vi "fpga4.vi"() -> ()   [LabVIEW 2015]
uses:
  <vilib>/LabVIEW Targets/FPGA/RIO/nicrio_985x_controls.llb/CAN_IO_Frame Cluster.ctl
  <vilib>/LabVIEW Targets/FPGA/RIO/nicrio_985x_controls.llb/CAN_IO_Frame Type.ctl
  <vilib>/rvi/Emulation/niFpgaGetClockAttributes.vi
  <vilib>/rvi/Emulation/niFpgaSctlEmulationGetInTimedLoop.vi
  <vilib>/rvi/Emulation/niFpgaEmulationReportErrorSimple.vi
  <vilib>/rvi/eio/common/nirviEmuTemplateMethod_errors.vi
  <vilib>/rvi/Emulation/niFpgaCriticalErrorInLSC.vi
  <vilib>/eio/EIONode/EIONode.xnode
  <vilib>/eio/EIOMethodNode/EIOMethodNode.xnode
panel:
  out "can 316":u8[](array[numeric])
  out "can 690":u8[](array[numeric])
  out "can 545":u8[](array[numeric])
  out "can 4F0":u8[](array[numeric])
  out "can 4B0":u8[](array[numeric])
  out "can 43F":u8[](array[numeric])
  out "can 392":u8[](array[numeric])
  out "can 329":u8[](array[numeric])
  out "can 220":u8[](array[numeric])
  out "can data":u32[](array[numeric])
  out "can 164":u8[](array[numeric])
  in  "Mod4/CAN1 input":T1={"timestamp high"=0, "timestamp low"=0, "identifier"=0, "type"=enum."Data Frame", "info A"=0, "info B"=0, "data length"=0, "data"=[0, 0, 0, 0, 0, 0, 0, 0]} {"identifier" format="%x"; "timestamp high" format="%08x"; "timestamp low" format="%08x"; "data" format="%.0x"}
  in  "send can":bool
  out "Mod4/CAN1 read":T1={"timestamp high"=0, "timestamp low"=0, "identifier"=0, "type"=enum."Data Frame", "info A"=0, "info B"=0, "data length"=0, "data"=[0, 0, 0, 0, 0, 0, 0, 0]} {"identifier" format="%x"; "timestamp high" format="%08x"; "timestamp low" format="%08x"; "data" format="%.0x"}
  out "can0 error out1":errorcluster
  out "can0 error out":errorcluster
  out "m 760":u8[](array[numeric])
  out "m 729":u8[](array[numeric])
  out "m 728":u8[](array[numeric])
  out "m 727":u8[](array[numeric])
  out "m 726":u8[](array[numeric])
  out "m 725":u8[](array[numeric])
  out "m 724":u8[](array[numeric])
  out "m 723":u8[](array[numeric])
  out "m 722":u8[](array[numeric])
  out "m 721":u8[](array[numeric])
  out "m 720":u8[](array[numeric])
  out "m 711":u8[](array[numeric])
  out "m 710":u8[](array[numeric])
  out "m 700":u8[](array[numeric])
  out "Mod4/CAN0":T1={"timestamp high"=0, "timestamp low"=0, "identifier"=0, "type"=enum."Data Frame", "info A"=0, "info B"=0, "data length"=0, "data"=[0, 0, 0, 0, 0, 0, 0, 0]} {"identifier" format="%x"; "timestamp high" format="%08x"; "timestamp low" format="%08x"; "data" format="%.0x"}
  out "brk enc":u8
  in  "baud rate":i32(ring)=4 items=["300", "1200", "2400", "4800", "9600", "14400", "19200", "28800", "38400", "57600", "115200", "230400"]
  in  "B Pwm":u16=1500
  in  "T Pwm":u16=1500
  in  "S Pwm 1":u16=1500
  in  "S Pwm 2":u16=1500
  out "Auto":bool
  out "Run":bool
  in  "Solenoid":bool
  in  "Buzz":bool
  out "T Lim":bool
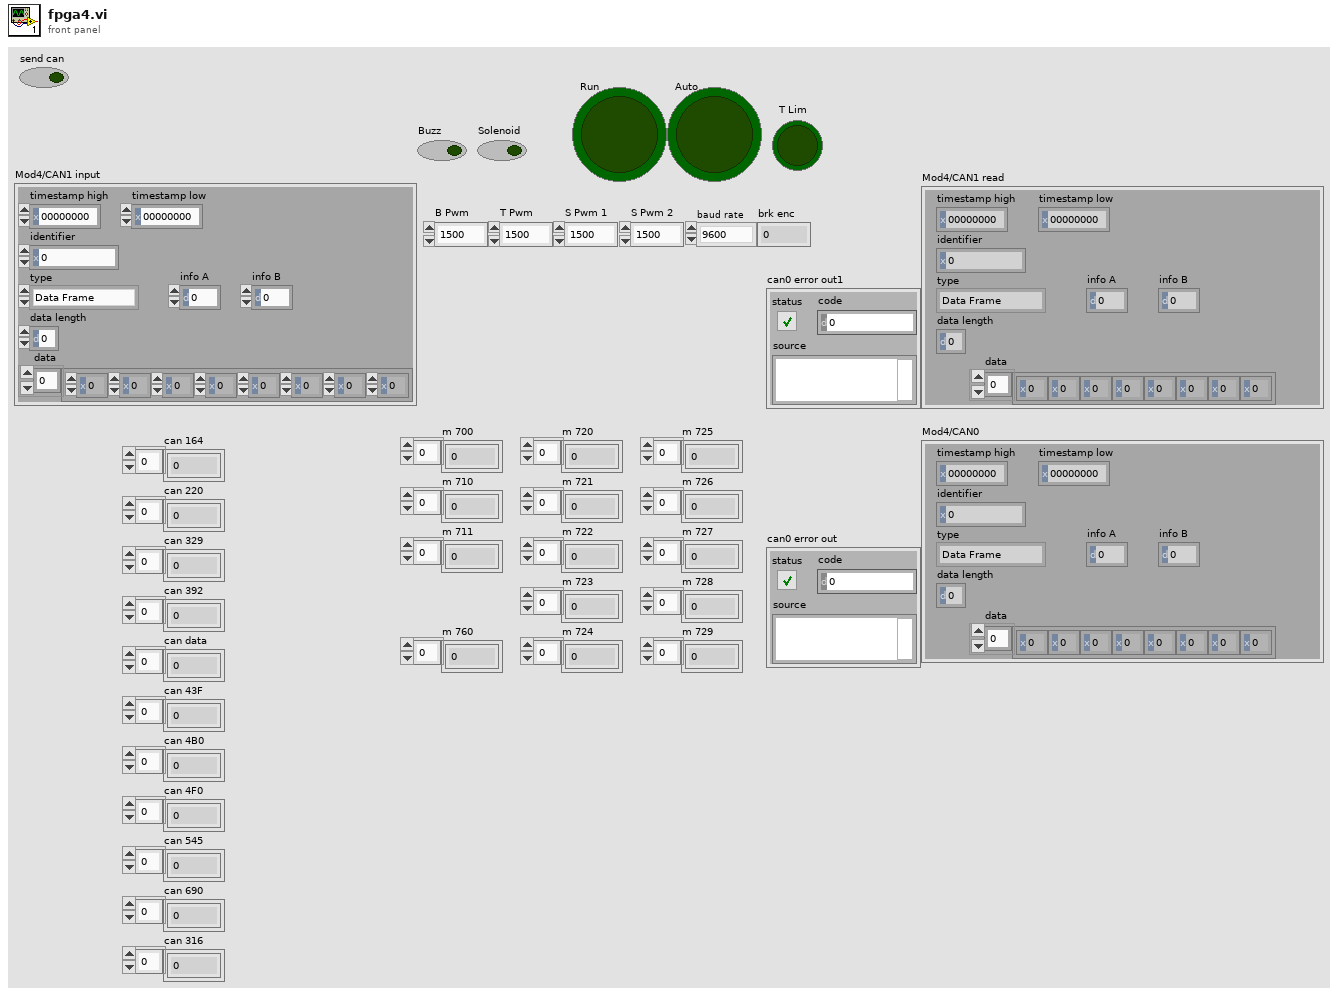
[diagram p1: front panel]
types:
  T1 = typedef "CAN_IO_Frame Cluster.ctl" = cluster{"timestamp high":u32, "timestamp low":u32, "identifier":u32, "type":T2, "info A":u8, "info B":u8, "data length":u8, "data":u8[]}
  T2 = typedef "CAN_IO_Frame Type.ctl" = enum8{"Data Frame", "Remote Frame", "(reserved)", "(reserved) ", "(reserved)  ", "(reserved)   ", "Bus Error", "Transceiver Fault"}
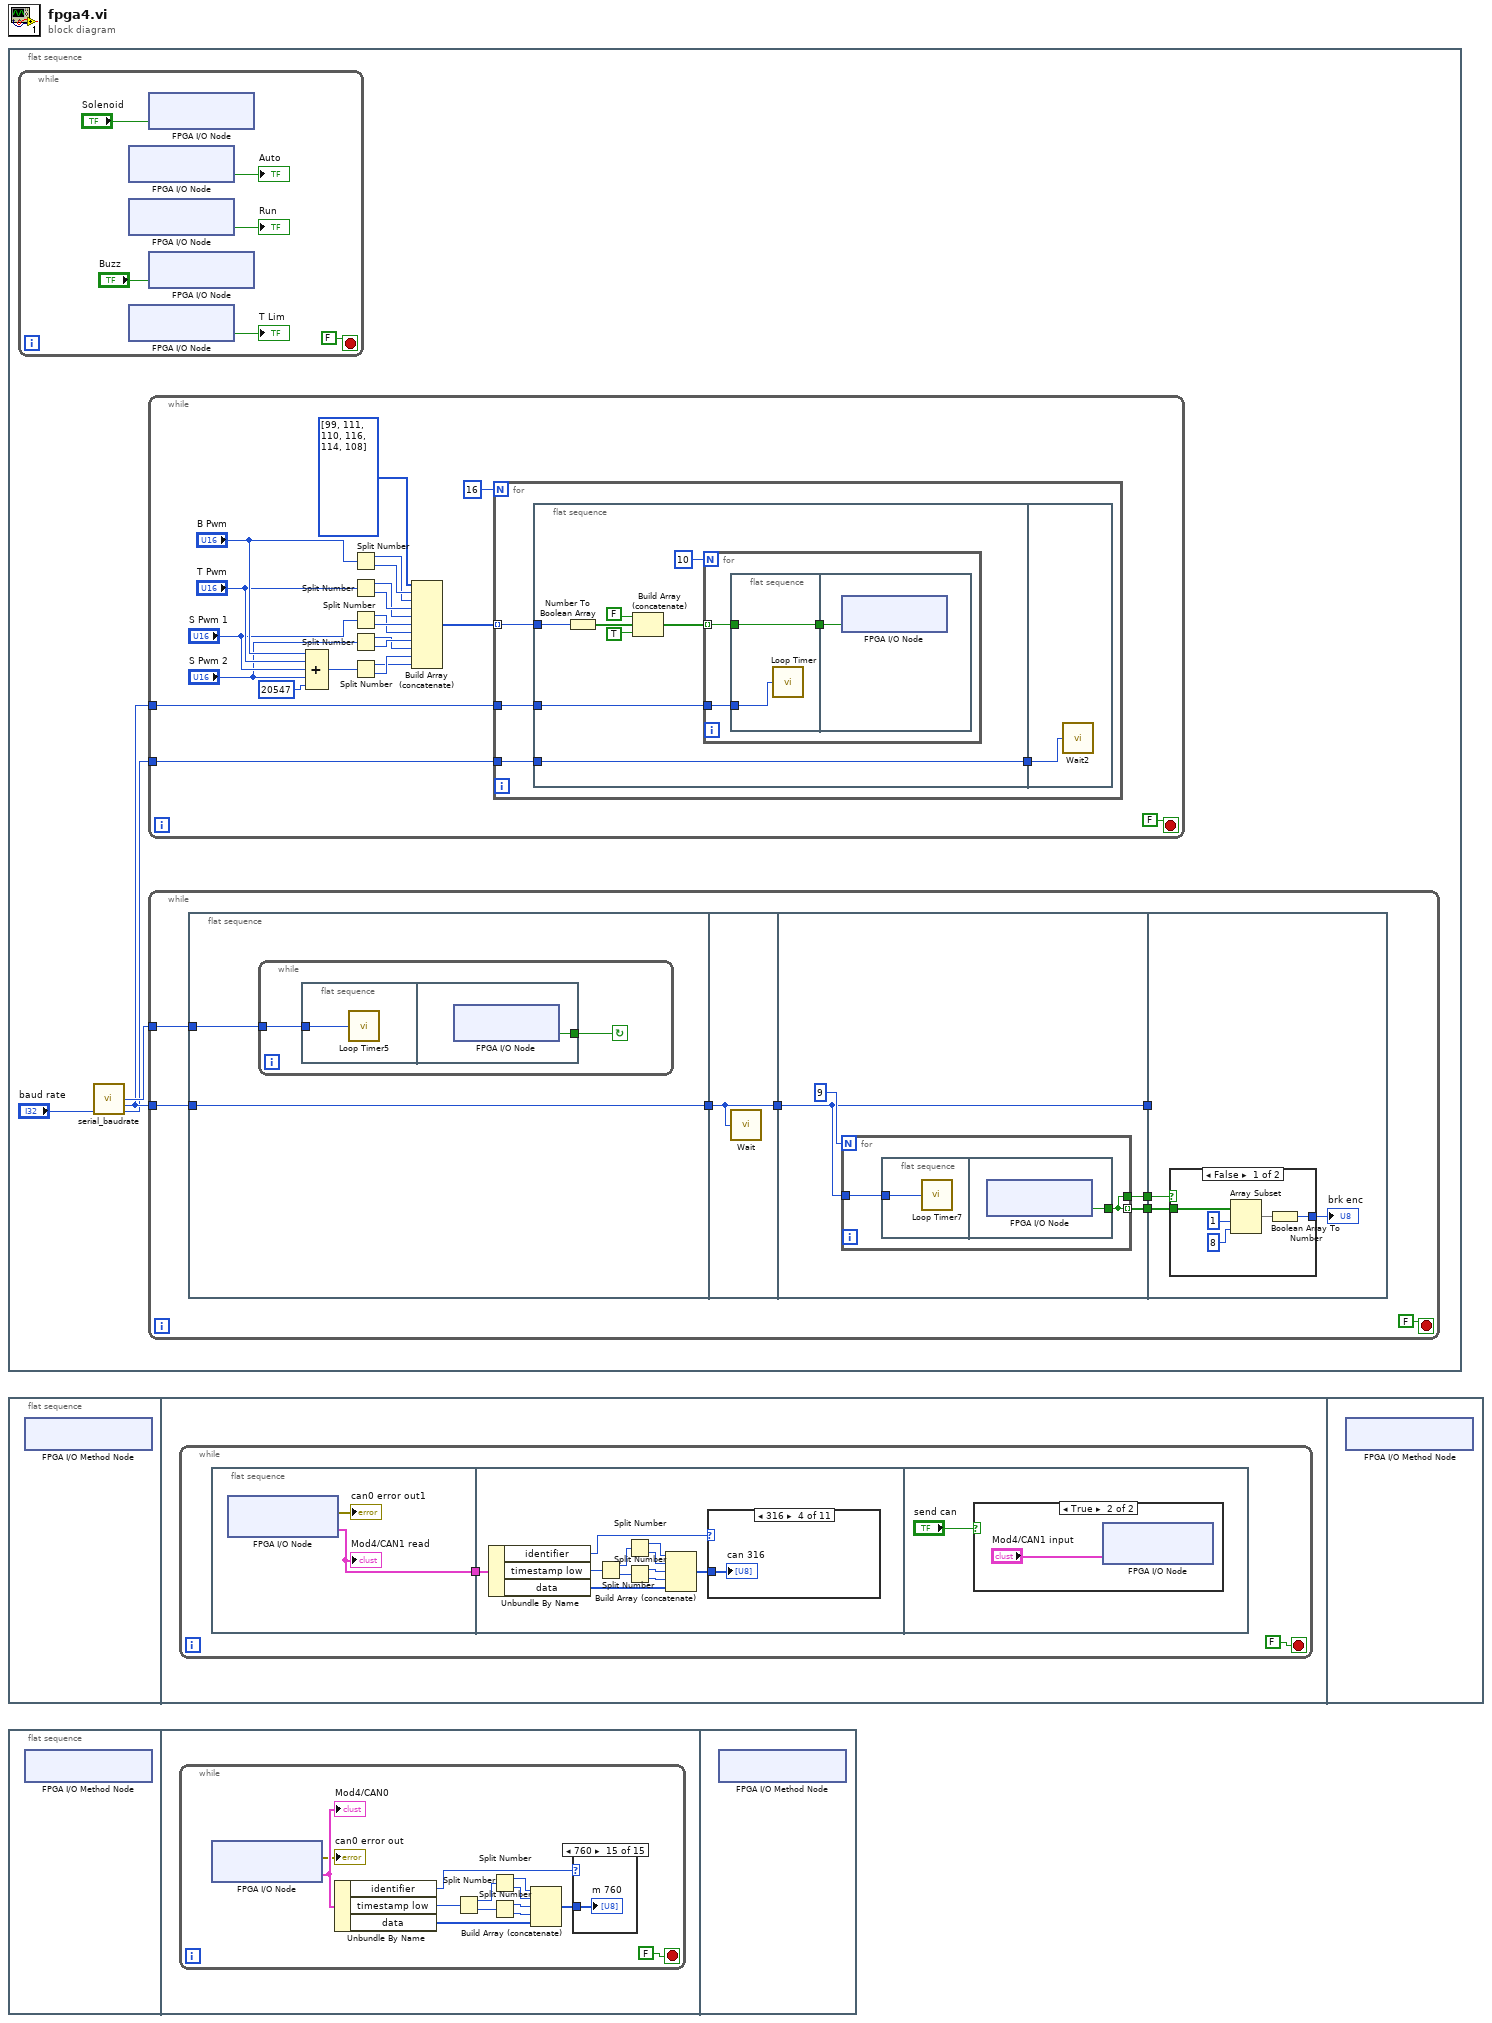
[diagram p0: block diagram]
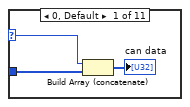
[diagram p2: hidden frame]
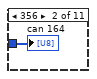
[diagram p3: hidden frame]
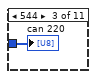
[diagram p4: hidden frame]
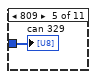
[diagram p5: hidden frame]
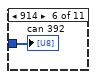
[diagram p6: hidden frame]
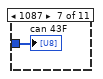
[diagram p7: hidden frame]
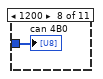
[diagram p8: hidden frame]
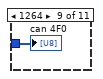
[diagram p9: hidden frame]
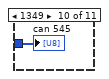
[diagram p10: hidden frame]
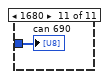
[diagram p11: hidden frame]
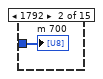
[diagram p14: hidden frame]
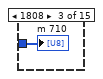
[diagram p15: hidden frame]
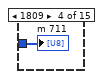
[diagram p16: hidden frame]
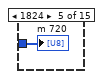
[diagram p17: hidden frame]
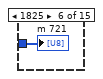
[diagram p18: hidden frame]
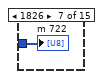
[diagram p19: hidden frame]
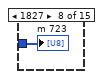
[diagram p20: hidden frame]
diagram:
  n1 = flat-sequence {
    frame #0 {
      n2 = while {
        stop <- FALSE stop-if-true
        n3 = xnode "FPGA I/O Node"() -> ("Mod3/DIO0"=→"Auto":bool)  [unwired: 1 in, 1 out]
        n4 = xnode "FPGA I/O Node"() -> ("Mod3/DIO3"=→"Run":bool)  [unwired: 1 in, 1 out]
        n5 = xnode "FPGA I/O Node"() -> ("Mod3/DIO2"=→"T Lim":bool)  [unwired: 1 in, 1 out]
        n6 = xnode "FPGA I/O Node"("Mod3/DIO4"="Solenoid") -> ()  [unwired: 1 in, 1 out]
        n7 = xnode "FPGA I/O Node"("Mod3/DIO5"="Buzz") -> ()  [unwired: 1 in, 1 out]
      }
      n8 = call "serial_baudrate.vi"("baud rate"="baud rate") -> ("tick/2 every bit"=w3:u32, "tick every bit"=w2:u32, "tick after stop bit"=w1:u32)  [unwired: 12 in]
      n9 = while {
        tunnel: w2 -> [w6]
        tunnel: w1 -> [w5]
        stop <- FALSE stop-if-true
        n10 = Compound Arithmetic op=ADD("B Pwm", "T Pwm", "S Pwm 1", "S Pwm 2", u16 20547 ("value")) -> (w11:u16)
        n11 = Split Number(x="B Pwm") -> (hi(x)=w24:u8, lo(x)=w25:u8)
        n12 = Split Number(x="T Pwm") -> (hi(x)=w22:u8, lo(x)=w23:u8)
        n13 = Split Number(x="S Pwm 1") -> (hi(x)=w20:u8, lo(x)=w21:u8)
        n14 = Split Number(x="S Pwm 2") -> (hi(x)=w18:u8, lo(x)=w19:u8)
        n15 = Split Number(x=w11) -> (hi(x)=w9:u8, lo(x)=w10:u8)
        n16 = Build Array (concatenate)(u8[] [99, 111, 110, 116, 114, 108] ("header"), w25, w24, w23, w22, w21, w20, w19, w18, w10, w9) -> (w8:u8[])
        n17 = for {
          N: 16 -> [_]
          tunnel: w8 -> [w30] mode=indexing
          tunnel: w6 -> [w29]
          tunnel: w5 -> [w28]
          n18 = flat-sequence {
            tunnel: w30 -> [w38]
            tunnel: w29 -> [w37]
            tunnel: w28 -> [w31]
            tunnel: [w31] -> w27
            tunnel: w27 -> [w45]
            frame #0 {
              n19 = Number To Boolean Array(number=w38) -> (Boolean array=w36:bool[])
              n20 = Build Array (concatenate)(FALSE, w36, TRUE) -> (w33:bool[])
              n21 = for {
                N: 10 -> [_]
                tunnel: w33 -> [w40] mode=indexing
                tunnel: w37 -> [w39]
                n22 = flat-sequence {
                  tunnel: [w43] -> w41
                  tunnel: w40 -> [w43]
                  tunnel: w39 -> [w42]
                  tunnel: w41 -> [w44]
                  frame #0 {
                    n23 = call "Loop Timer"("Count(Ticks)"=w42) -> ()  [unwired: 1 out]
                  }
                  frame #1 {
                    n24 = xnode "FPGA I/O Node"("Mod3/DIO6"=w44) -> ()  [unwired: 1 in, 1 out]
                  }
                }
              }
            }
            frame #1 {
              n25 = call "Wait2"("Count(Ticks)"=w45) -> ()  [unwired: 1 out]
            }
          }
        }
      }
      n26 = while {
        tunnel: w2 -> [w48]
        tunnel: w3 -> [w47]
        stop <- FALSE stop-if-true
        n27 = flat-sequence {
          tunnel: w47 -> [w55]
          tunnel: [w54] -> w53
          tunnel: w48 -> [w54]
          tunnel: w53 -> [w60]
          tunnel: [w60] -> w52
          tunnel: [w63] -> w51
          tunnel: [w62] -> w50
          tunnel: w52 -> [w61]
          tunnel: [w61] -> w49
          tunnel: w51 -> [w69]
          tunnel: w50 -> [w71]
          tunnel: w49 -> [_]
          frame #0 {
            n28 = while {
              tunnel: w55 -> [w56]
              stop <- w57 continue-if-true
              n29 = flat-sequence {
                tunnel: w56 -> [w58]
                tunnel: [w59] -> w57
                frame #0 {
                  n30 = call "Loop Timer5"("Count(Ticks)"=w58) -> ()  [unwired: 1 out]
                }
                frame #1 {
                  n31 = xnode "FPGA I/O Node"() -> ("Mod3/DIO1"=w59:bool)  [unwired: 1 in, 1 out]
                }
              }
            }
          }
          frame #1 {
            n32 = call "Wait"("Count(Ticks)"=w60) -> ()  [unwired: 1 out]
          }
          frame #2 {
            n33 = for {
              N: 9 -> [_]
              tunnel: [w66] -> w62 mode=indexing
              tunnel: [w66] -> w63
              tunnel: w61 -> [w65]
              n34 = flat-sequence {
                tunnel: w65 -> [w67]
                tunnel: [w68] -> w66
                frame #0 {
                  n35 = call "Loop Timer7"("Count(Ticks)"=w67) -> ()  [unwired: 1 out]
                }
                frame #1 {
                  n36 = xnode "FPGA I/O Node"() -> ("Mod3/DIO1"=w68:bool)  [unwired: 1 in, 1 out]
                }
              }
            }
          }
          frame #3 {
            n37 = case shown="False" w69 {
              tunnel: w71 -> [w73 w78]
              tunnel: [w74 w79] -> w70
              frame False {
                n38 = Array Subset(array=w73, index=1, length=8) -> (w72:bool[])
                n39 = Boolean Array To Number(Boolean array=w72) -> (number=w74:u8)
              }
              frame True {
                n40 = Array Subset(array=w78, index=0, length=8) -> (w77:bool[])
                n41 = Boolean Array To Number(Boolean array=w77) -> (number=w79:u8)
              }
            }
            "brk enc" <- w70
          }
        }
      }
    }
  }
  n42 = flat-sequence {
    frame #0 {
      n43 = xnode "FPGA I/O Method Node"() -> ()  [unwired: 1 in, 1 out]
    }
    frame #1 {
      n44 = while {
        stop <- FALSE stop-if-true
        n45 = flat-sequence {
          tunnel: [w90] -> w88
          tunnel: w88 -> [w102]
          frame #0 {
            n46 = xnode "FPGA I/O Node"() -> ("error out"=→"can0 error out1":errorcluster, "Mod4/CAN1"=w90:T1)  [unwired: 2 in, 1 out]
            "Mod4/CAN1 read" <- w90
          }
          frame #1 {
            n47 = Unbundle By Name(w102) -> ("identifier"=w101:u32, "timestamp low"=w95:u32, "data"=w94:u8[])
            n48 = Split Number(x=w95) -> (hi(x)=w96:u16, lo(x)=w97:u16)
            n49 = Split Number(x=w96) -> (hi(x)=w92:u8, lo(x)=w98:u8)
            n50 = Split Number(x=w97) -> (hi(x)=w99:u8, lo(x)=w100:u8)
            n51 = Build Array (concatenate)(w92, w98, w99, w100, w94) -> (w93:u8[])
            n52 = case shown="316" w101 {
              selector: w101 -> [w105 _ _ _ _ _ _ _ _ _ _]
              tunnel: w93 -> [w104 w106 w107 w108 w109 w110 w111 w112 w113 w114 w115]
              frame 0, Default {
                n53 = Build Array (concatenate)(w105, w104) -> (→"can data":u32[])
              }
              frame 356 {
                "can 164" <- w106
              }
              frame 544 {
                "can 220" <- w107
              }
              frame 790 {
                "can 316" <- w108
              }
              frame 809 {
                "can 329" <- w109
              }
              frame 914 {
                "can 392" <- w110
              }
              frame 1087 {
                "can 43F" <- w111
              }
              frame 1200 {
                "can 4B0" <- w112
              }
              frame 1264 {
                "can 4F0" <- w113
              }
              frame 1349 {
                "can 545" <- w114
              }
              frame 1680 {
                "can 690" <- w115
              }
            }
          }
          frame #2 {
            n54 = case shown="True" "send can" {
              frame False {
              }
              frame True {
                n55 = xnode "FPGA I/O Node"("Mod4/CAN1"="Mod4/CAN1 input") -> ()  [unwired: 2 in, 2 out]
              }
            }
          }
        }
      }
    }
    frame #2 {
      n56 = xnode "FPGA I/O Method Node"() -> ()  [unwired: 1 in, 1 out]
    }
  }
  n57 = flat-sequence {
    frame #0 {
      n58 = xnode "FPGA I/O Method Node"() -> ()  [unwired: 1 in, 1 out]
    }
    frame #1 {
      n59 = while {
        stop <- FALSE stop-if-true
        n60 = xnode "FPGA I/O Node"() -> ("error out"=→"can0 error out":errorcluster, "Mod4/CAN0"=w129:T1)  [unwired: 2 in, 1 out]
        "Mod4/CAN0" <- w129
        n61 = Unbundle By Name(w129) -> ("identifier"=w128:u32, "timestamp low"=w127:u32, "data"=w120:u8[])
        n62 = Split Number(x=w127) -> (hi(x)=w126:u16, lo(x)=w125:u16)
        n63 = Split Number(x=w126) -> (hi(x)=w124:u8, lo(x)=w123:u8)
        n64 = Split Number(x=w125) -> (hi(x)=w122:u8, lo(x)=w121:u8)
        n65 = Build Array (concatenate)(w124, w123, w122, w121, w120) -> (w119:u8[])
        n66 = case shown="760" w128 {
          tunnel: w119 -> [_ w131 w132 w133 w134 w135 w136 w137 w138 w139 w140 w141 w142 w143 w144]
          frame 0, Default {
          }
          frame 1792 {
            "m 700" <- w131
          }
          frame 1808 {
            "m 710" <- w132
          }
          frame 1809 {
            "m 711" <- w133
          }
          frame 1824 {
            "m 720" <- w134
          }
          frame 1825 {
            "m 721" <- w135
          }
          frame 1826 {
            "m 722" <- w136
          }
          frame 1827 {
            "m 723" <- w137
          }
          frame 1828 {
            "m 724" <- w138
          }
          frame 1829 {
            "m 725" <- w139
          }
          frame 1830 {
            "m 726" <- w140
          }
          frame 1831 {
            "m 727" <- w141
          }
          frame 1832 {
            "m 728" <- w142
          }
          frame 1833 {
            "m 729" <- w143
          }
          frame 1888 {
            "m 760" <- w144
          }
        }
      }
    }
    frame #2 {
      n67 = xnode "FPGA I/O Method Node"() -> ()  [unwired: 1 in, 1 out]
    }
  }
